vi "6. import Config.ini with __include section.vi"() -> (3 "RS232_Device Config":T1={"Resource"="com5", "baud rate"=115200, "data bits"=8, "parity"=enum."Odd", "stop bits"=10})   [LabVIEW 2017]
uses:
  f65b758a-57a2-4ff6-b8fb-5289b55a65bc.vi
  f65b758a-57a2-4ff6-b8fb-5289b55a65bc.vi/99de0c97-112a-4c86-9094-c187659127e1.vi
  <userlib>/_NEVSTOP/Communicable State Machine(CSM)/Utility/Build Error Cluster.vi
  <vilib>/Utility/Data Type/Get Type Information.vi
  <userlib>/_NEVSTOP/Communicable State Machine(CSM)/addons/API-String-Arugments-Support/_Support/Data To SingleElementsArray_csm.vi
  <userlib>/_NEVSTOP/Communicable State Machine(CSM)/addons/API-String-Arugments-Support/_Support/Data To API String Arguments.vi
  INI-Static-Variable-Support/_Support/Parse Used Session and Name.vi
  INI-Static-Variable-Support/_Support/INI-FGV(lvlibp).vi
  INI-Static-Variable-Support/_Support/Populate String with INI Variable.vi
  <userlib>/_NEVSTOP/Communicable State Machine(CSM)/addons/API-String-Arugments-Support/_Support/Convert API String Arguments to Data(variant).vi
  <userlib>/_NEVSTOP/Communicable State Machine(CSM)/addons/API-String-Arugments-Support/_Support/SingleElementsArray To Data_csm.vi
  INI-Static-Variable-Support/INI-Static-Variable-Support.lvlib
panel:
  out "All Config Files":path[](array[path])
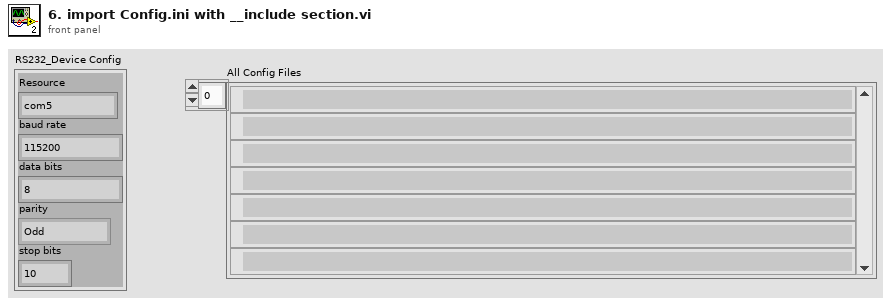
[diagram p1: front panel]
types:
  T1 = cluster{"Resource":string, "baud rate":u32, "data bits":u16, "parity":enum16{"None", "Odd", "Even", "Mark", "Space"}, "stop bits":u16}
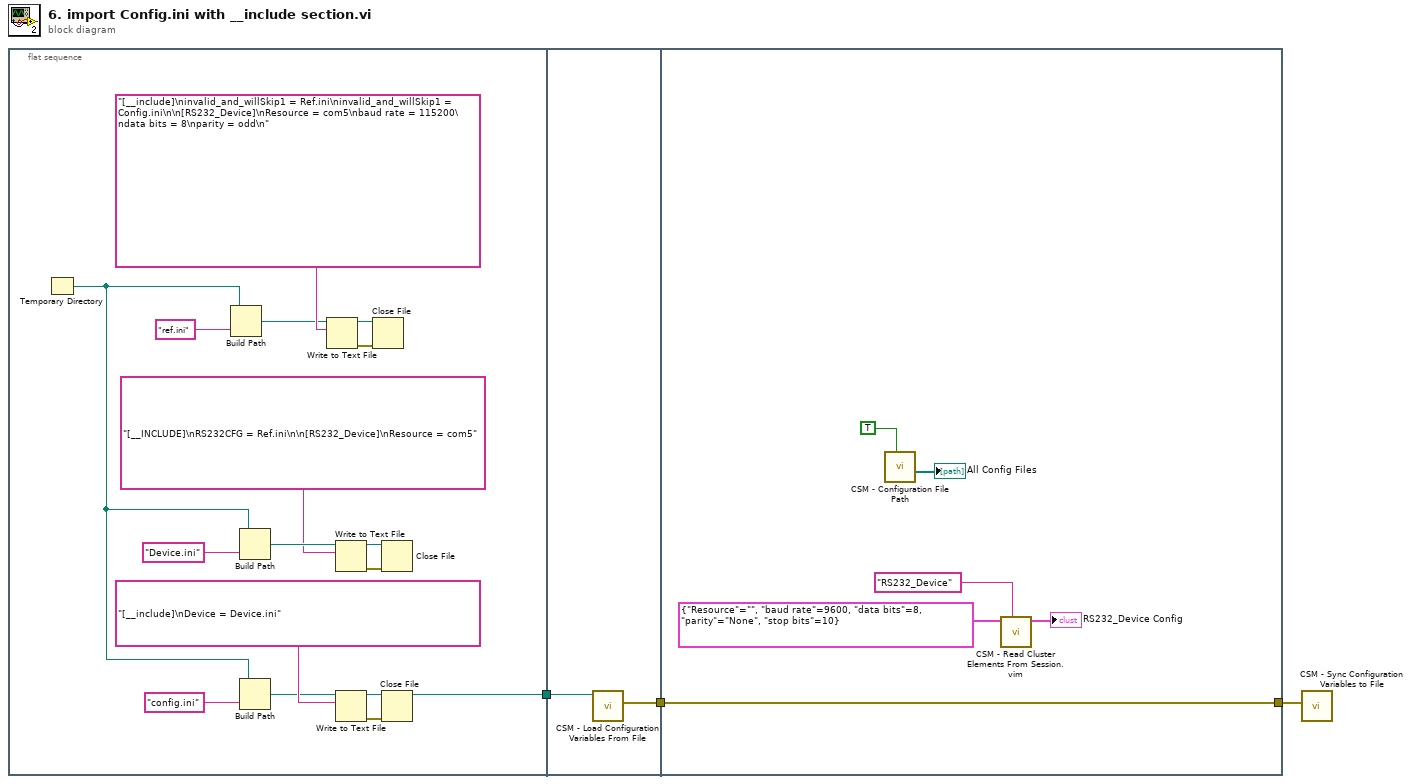
[diagram p0: block diagram]
diagram:
  n1 = flat-sequence {
    tunnel: [w5] -> w1
    tunnel: [w22] -> w3
    tunnel: w1 -> [w21]
    tunnel: w3 -> [w23]
    tunnel: [w23] -> w2
    frame #0 {
      n2 = Temporary Directory() -> (w4:path)
      n3 = Build Path(base path=w4, name or relative path="ref.ini" ("Temporary File Extension (tmp)")) -> (appended path=w16:path)
      n4 = Build Path(base path=w4, name or relative path="Device.ini" ("Temporary File Extension (tmp)")) -> (appended path=w15:path)
      n5 = Build Path(base path=w4, name or relative path="config.ini" ("Temporary File Extension (tmp)")) -> (appended path=w6:path)
      n6 = Write to Text File(file (use dialog)=w16, text="[__include]\ninvalid_and_willSkip1 = Ref.ini\ninvalid_and_willSkip1 = Config.ini\n\n[RS232_Device]\nResource = com5\nbaud rate = 115200\ndata bits = 8\nparity = odd\n") -> (refnum out=w19:refnum<file>, error out=w20:errorcluster)  [unwired: 2 in, 1 out]
      n7 = Write to Text File(file (use dialog)=w15, text="[__INCLUDE]\nRS232CFG = Ref.ini\n\n[RS232_Device]\nResource = com5") -> (refnum out=w13:refnum<file>, error out=w12:errorcluster)  [unwired: 2 in, 1 out]
      n8 = Write to Text File(file (use dialog)=w6, text="[__include]\nDevice = Device.ini") -> (refnum out=w8:refnum<file>, error out=w9:errorcluster)  [unwired: 2 in, 1 out]
      n9 = Close File(refnum=w19, error in=w20) -> ()  [unwired: 2 out]
      n10 = Close File(refnum=w13, error in=w12) -> ()  [unwired: 2 out]
      n11 = Close File(refnum=w8, error in=w9) -> (path=w5:path)  [unwired: 1 out]
    }
    frame #1 {
      n12 = call "CSM - Load Configuration Variables From File.vi"("Path"=w21) -> ("error out"=w22:errorcluster)  [unwired: 8 in]
    }
    frame #2 {
      n13 = call "CSM - Configuration File Path.vi"("Include All Paths?(F)"=TRUE) -> ("All Config Files"=→"All Config Files":path[])  [unwired: 6 in, 2 out]
      n14 = call "CSM - Read Cluster Elements From Session.vim"("Section Name(\"\" as Default)"="RS232_Device" ("Section Name(\"\" as Default)"), "Cluster"=T1 {"Resource"="", "baud rate"=9600, "data bits"=8, "parity"=enum."None", "stop bits"=10}) -> ("Cluster out"=→"RS232_Device Config":T1)  [unwired: 6 in, 1 out]
    }
  }
  n15 = call "CSM - Sync Configuration Variables to File.vi"("error in (no error)"=w2) -> ()  [unwired: 8 in, 1 out]
